vi "InsertFailTransactionReplyOnError.vi"(8 "Error In":errorcluster, 11 "Replies In":string[](array[string])) -> (0 "Error Out":errorcluster, 3 "Replies Out":string[](array[string]))   [LabVIEW 2020, in "NI_XNodeSupport.lvlib"]
uses:
  NI_XNodeSupport.lvlib
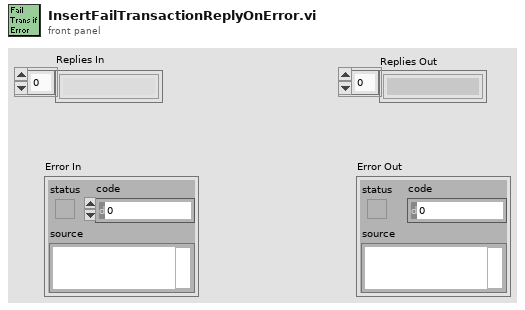
[diagram p1: front panel]
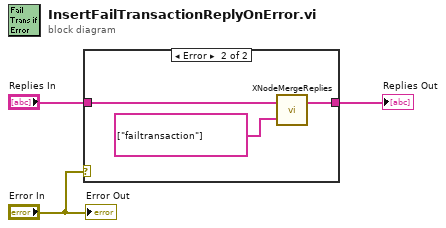
[diagram p0: block diagram]
diagram:
  n1 = case shown="Error" "Error In" {
    tunnel: "Replies In" -> [w4 w7]
    tunnel: [w4 w6] -> w2
    frame No Error {
    }
    frame Error {
      n2 = call "XNodeMergeReplies.vi"("New Replies"=string[] ["failtransaction"], "Old Replies"=w7) -> ("Merged Replies"=w6:string[])
    }
  }
  "Replies Out" <- w2
  "Error Out" <- "Error In"
